vi "Grab images from pco.edge or pco.pixelfly USB.vi"() -> ()   [LabVIEW 2012]
doc: "A short program to demonstrate the fundamentals of control and image acquision with the pco.camera series. The program records a sequence of images, with \"live\" updating, until the \"StopRecording\" button is pressed. Use ctrl-H for more help on the individual controls and indicators.\n\nCopyright 2004, 2010 The Cooke Corporation."
panel:
  out "bClose":bool
  in  "Quit":bool
  out "BufNr1":i16
  out "BufNr0":i16
  in  "bUseBuffer1":bool
  in  "bUseBuffer0":bool
  in  "ROIX1":u16=1 min=1
  in  "ROIY1":u16=1 min=1
  in  "ROIY0":u16=1 min=1
  in  "ROIX0":u16=1 min=1
  out "Bits/pixel":u16
  in  "Record":bool
  in  "DelayTimeBase":u16(ring)=2 items=["nanoseconds", "microseconds", "milliseconds"]
  in  "ExposureTimeBase":u16(ring)=2 items=["nanoseconds", "microseconds", "milliseconds"]
  in  "Exposure":u32=10
  in  "Delay":u32
  in  "Rate":i32(ring) items=["12500000", "25000000"]
  out "Image":u16[][](graph)
  in  "TriggerMode":u16(ring) items=["Auto", "Software", "External sequence start ", "External exposure control"]
  # "A short program to demonstrate the fundamentals of control and image acquision with the pco.camera series. The program records a sequence of images, with \"live\" updating, until the \"StopRecording\" button is pressed.  Use ctrl-H for more help on the individual controls and indicators."
  # "pco.labview"
  # "1) Setup camera:"
  # "2) Record  images:"
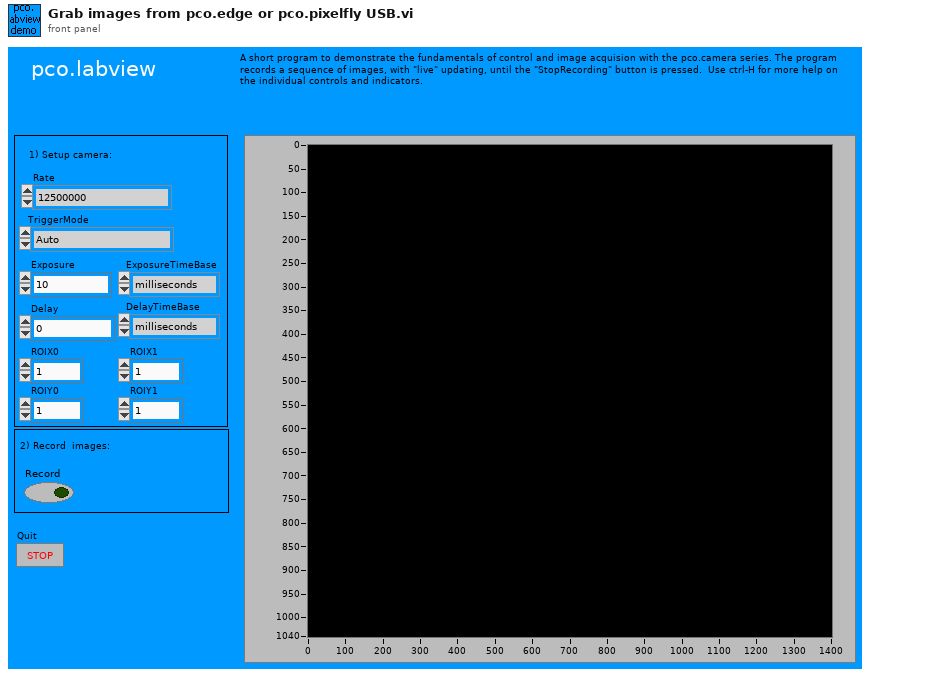
[diagram p1: front panel]
types:
  T1 = cluster{"SSize":u16, "CamType":u16, "CamsSubType":u16, "SerialNumber":u32, "HWVersion":u32, "FWVersion ":u32, "InterfaceType":u16, "HardwareVersions":cluster{"Board":u16, cluster{"string":string, "BatchNumber":u16, "MinorRevision":u8, "MajorRevision":u8, "Variant":u16}[]}, "FirmwareVersions":cluster{"DeviceNum":u16, cluster{"string":string, "MinorRevision":u8, "MajorRevision":u8, "Variant":u16}[]}}
  T2 = cluster{"Size":u16, "SensorTypeDESC":u16, "SensorSubtypeDESC":u16, "MaxHorizontalResStdDESC":u16, "MaxVerticalResStdDESC":u16, "MaxHorizontalResExtDESC":u16, "MaxVerticalResExtDESC":u16, "DynResDESC":u16, "MaxBinHorzDESC":u16, "BinHorzStepDESC":bool, "MaxBinVertDESC":u16, "BinVertStepDESC":bool, "ROIHorzStepDESC":u16, "ROIVertStepDESC":u16, "NumADCDESC":u16, "IRDESC":bool, "MinDelayDESC":u32, "MaxDelayDESC":u32, "MinDelayStepDESC":u32, "MinExpoDESC":u32, "MaxExpoDESC":u32, "MinExpoStepDESC":u32, "MinDelayIRDESC":u32, "MaxDelayIRDESC":u32, "MinExpoIRDESC":u32, "MaxExpoIRDESC":u32, "TimeTableDESC":bool, "DoubleImageDESC":bool, "MinCoolSetDESC":i16, "MaxCoolSetDESC":i16, "MDefaultCoolSetDESC":i16, "PowerDownModeDESC":bool, "OffsetRegDESC":bool, "ColorPattern":cluster{"UpperLeftColor":u8, "UpperRightColor":u8, "LowerLeftColor":u8, "LowerRightColor":u8}, "PatternTypeDESC":bool, "PixelRates":u32[], "CoversionFactors":u16[], "Reserved":u32[], "GeneralCapabilities":u32, "GeneralCapabilities 2":u32, "Min Size Hor":u16, "Min Size Vert":u16, "Ext Synch Freq":u32[], "Cooling Setpoints":i16[], "Soft ROI Hor Step":u16, "Soft ROI Vert Step":u16}
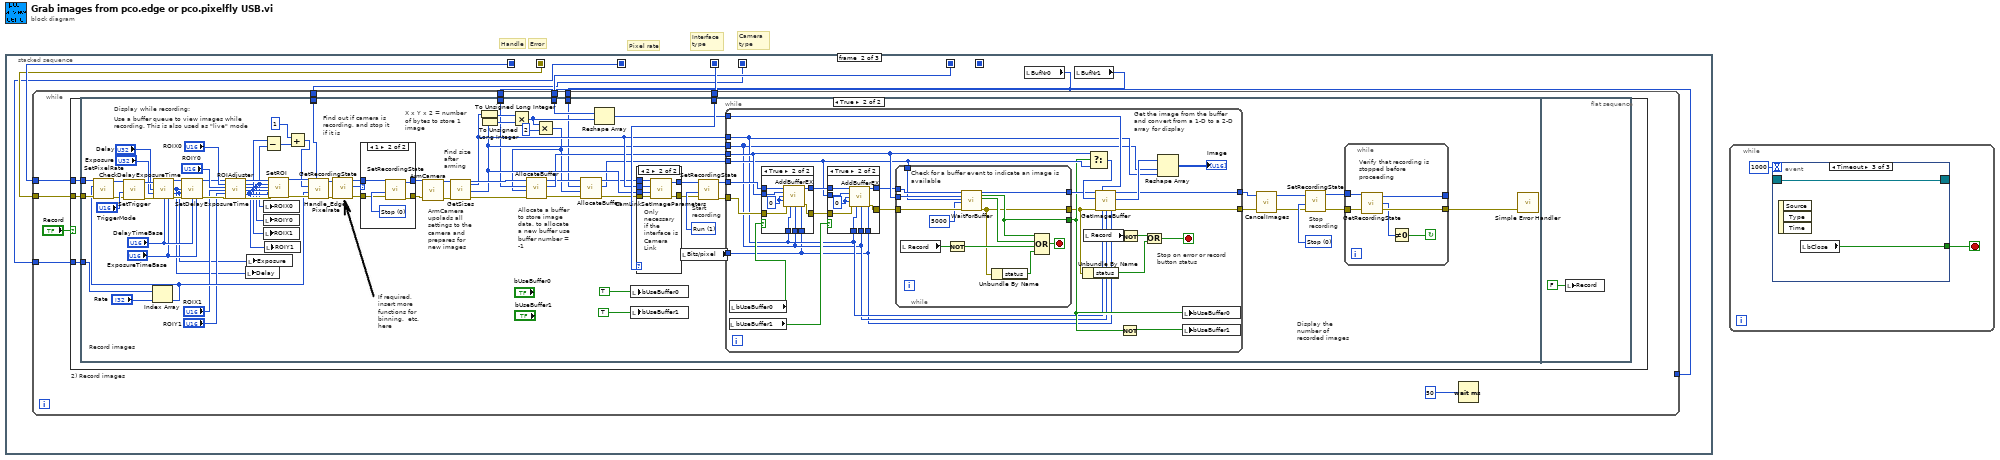
[diagram p0: block diagram]
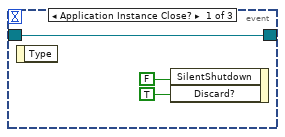
[diagram p2: hidden frame]
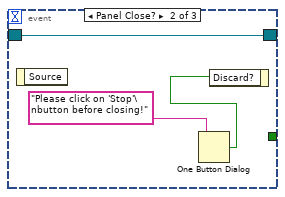
[diagram p3: hidden frame]
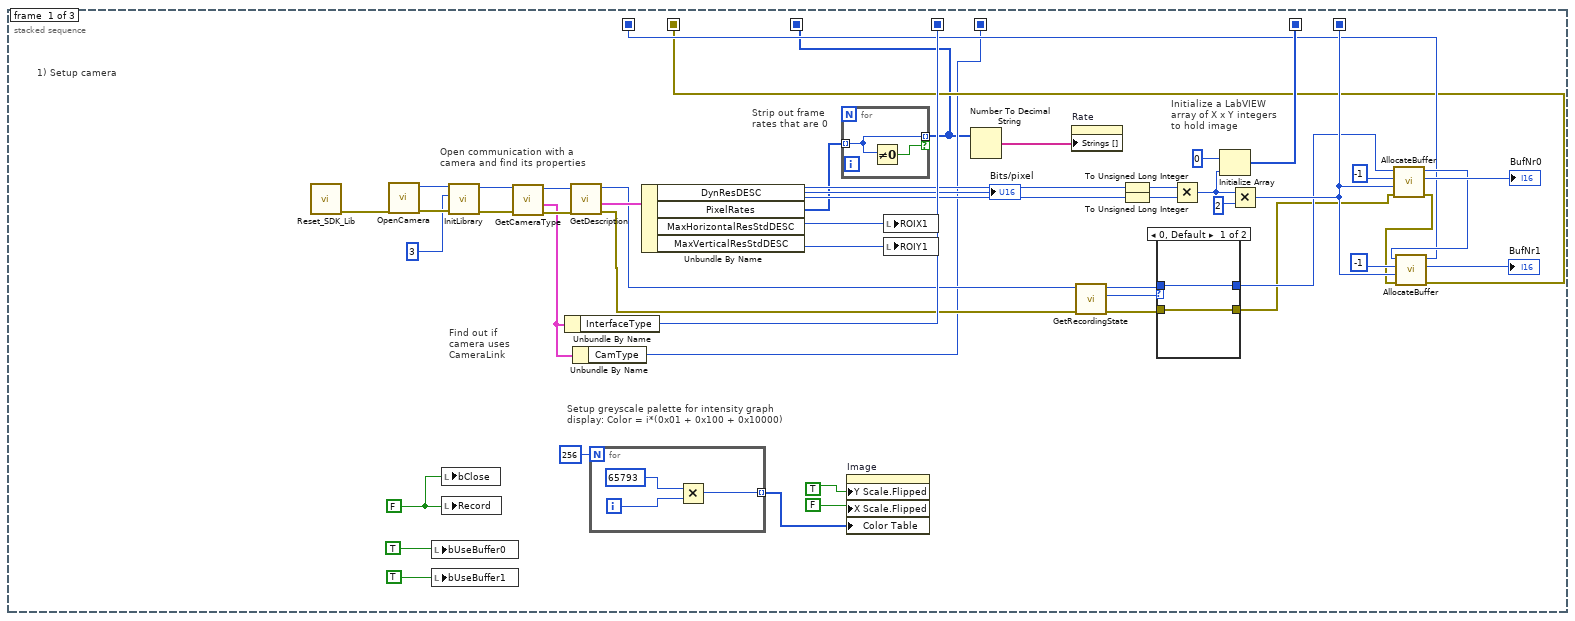
[diagram p4: hidden frame]
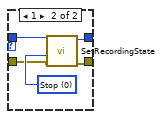
[diagram p5: hidden frame]
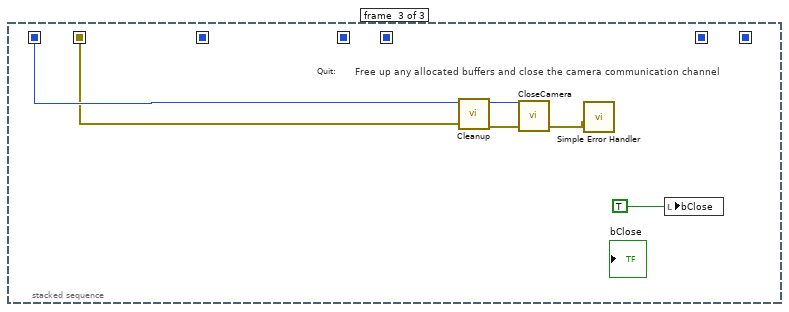
[diagram p11: hidden frame]
diagram:
  # "Camera type"
  # "Interface type"
  # "Error"
  # "Handle"
  # "Pixel rate"
  n1 = stacked-sequence {
    seq-local: [w41 _ _] -> [_ w64 _]
    seq-local: [w29 _ _] -> [_ _ _]
    seq-local: [w9 _ _] -> [_ w67 w253]
    seq-local: [w8 _ _] -> [_ w66 w252]
    seq-local: [w36 _ _] -> [_ w65 _]
    seq-local: [w1 _ _] -> [_ w61 _]
    seq-local: [w3 _ _] -> [_ w60 _]
    frame #0 {
      w23 = FALSE ("stop")
      # "Strip out frame rates that are 0"
      # "1) Setup camera"
      # "Find out if camera uses CameraLink"
      # "Setup greyscale palette for intensity graph display: Color = i*(0x01 + 0x100 + 0x10000)"
      # "Initialize a LabVIEW array of X x Y integers to hold image"
      # "Open communication with a camera and find its properties"
      n2 = call "Reset_SDK_Lib.vi"() -> ("ErrorOut"=w5:errorcluster)  [unwired: 11 in]
      n3 = call "OpenCamera.vi"("ErrorIn"=w5) -> ("ErrorOut"=w20:errorcluster, "Handle out"=w21:u64)  [unwired: 3 in, 2 out]
      n4 = local write "bUseBuffer0"(TRUE) -> ()
      n5 = local write "bUseBuffer1"(TRUE) -> ()
      n6 = local write "bClose"(w23) -> ()
      n7 = local write "Record"(w23) -> ()
      n8 = call "InitLibrary.vi"("error in (no error)"=w20, "InterfaceType"=u32 3, "ph"=w21) -> ("error out"=w19:errorcluster, "hout"=w18:u64)  [unwired: 7 in]
      n9 = call "GetCameraType.vi"("ph"=w18, "error in (no error)"=w19) -> ("hout"=w38:u64, "CameraType"=w4:T1, "error out"=w37:errorcluster)  [unwired: 1 in, 1 out]
      n10 = Unbundle By Name(w4) -> ("InterfaceType"=w36:u16)
      n11 = call "GetDescription.vi"("ErrorIn"=w37, "ph"=w38) -> ("ErrorOut"=w15:errorcluster, "Description"=w40:T2, "hout"=w14:u64)  [unwired: 2 in, 1 out]
      n12 = Unbundle By Name(w4) -> ("CamType"=w3:u16)
      n13 = for {
        N: 256 -> [_]
        tunnel: [w57] -> w44 mode=indexing
        i -> [w58]
        n14 = Multiply(x=65793, y=w58) -> (x*y=w57:i32)
      }
      n15 = Unbundle By Name(w40) -> ("DynResDESC"=→"Bits/pixel":u16, "PixelRates"=w2:u32[], "MaxHorizontalResStdDESC"=w34:u16, "MaxVerticalResStdDESC"=w33:u16)
      n16 = for {
        tunnel: w2 -> [w48] mode=indexing
        tunnel: [w48] -> w1 mode=indexing if=w49
        n17 = Not Equal To 0?(x=w48) -> (x != 0?=w49:bool)
      }
      n18 = property on="Image" class="IntGraph (strict)"("Y Scale.Flipped"=TRUE, "X Scale.Flipped"=FALSE, "Color Table"=w44) -> ()  [unwired: 2 in, 2 out]
      n19 = local write "ROIX1"(w34) -> ()
      n20 = local write "ROIY1"(w33) -> ()
      n21 = Number To Decimal String(number=w1) -> (decimal integer string=w22:string[])  [unwired: 1 in]
      n22 = property on="Rate" class="Ring (strict)"("Strings []"=w22) -> ()  [unwired: 2 in, 2 out]
      n23 = call "GetRecordingState.vi"("ErrorIn"=w15, "ph"=w14) -> ("ErrorOut"=w12:errorcluster, "Error"=w6:i32, "hout"=w13:u64)  [unwired: 2 in, 1 out]
      n24 = To Unsigned Long Integer(number=w34) -> (unsigned 32bit integer=w31:u32)
      n25 = To Unsigned Long Integer(number=w33) -> (unsigned 32bit integer=w30:u32)
      n26 = case shown="0, Default" w6 {
        tunnel: w13 -> [w51 w55]
        tunnel: w12 -> [w50 w54]
        tunnel: [w51 w53] -> w11
        tunnel: [w50 w52] -> w7
        frame 0, Default {
        }
        frame 1 {
          w56 = u16 0 items=["Stop", "Run"] ("RecordingState")
          n27 = call "SetRecordingState.vi"("ErrorIn"=w54, "RecordingState"=w56, "ph"=w55) -> ("ErrorOut"=w52:errorcluster, "hout"=w53:u64)  [unwired: 2 in, 1 out]
        }
      }
      n28 = Multiply(x=w31, y=w30) -> (x*y=w42:u32)
      n29 = Initialize Array(u16 0 ("Element Data"), w42) -> (w41:u16[])
      n30 = Multiply(x=w42, y=u32 2) -> (x*y=w29:u32)
      n31 = call "AllocateBuffer.vi"("error in (no error)"=w7, "Size"=w29, "BufNr"=i16 -1, "ph"=w11) -> ("error out"=w16:errorcluster, "BufNrOut"=→"BufNr0":i16, "hout"=w10:u64)  [unwired: 2 in, 3 out]
      n32 = call "AllocateBuffer.vi"("error in (no error)"=w16, "Size"=w29, "BufNr"=i16 -1, "ph"=w10) -> ("error out"=w8:errorcluster, "BufNrOut"=→"BufNr1":i16, "hout"=w9:u64)  [unwired: 2 in, 3 out]
    }
    frame #1 {
      n33 = local read "BufNr0"() -> (w63:i16)
      n34 = local read "BufNr1"() -> (w62:i16)
      n35 = while {
        tunnel: w63 -> [_]
        tunnel: w63 -> [w73]
        tunnel: w64 -> [w75]
        tunnel: w65 -> [w76]
        tunnel: w66 -> [w74]
        tunnel: w67 -> [w71]
        tunnel: w62 -> [w72]
        tunnel: w61 -> [w69]
        tunnel: w60 -> [w68]
        stop <- "Quit" stop-if-true
        n36 = case "2) Record images" shown="True" "Record" {
          tunnel: w71 -> [_ w86]
          tunnel: w74 -> [_ w85]
          tunnel: w76 -> [_ w84]
          tunnel: w75 -> [_ w83]
          tunnel: w73 -> [_ w82]
          tunnel: w72 -> [_ w81]
          tunnel: w69 -> [_ w80]
          tunnel: w68 -> [_ w79]
          frame False {
          }
          frame True {
            n37 = flat-sequence {
              tunnel: w86 -> [w151]
              tunnel: w85 -> [w150]
              tunnel: w84 -> [w148]
              tunnel: w83 -> [w146]
              tunnel: w82 -> [w137]
              tunnel: w81 -> [w131]
              tunnel: w80 -> [w118]
              tunnel: w79 -> [w109]
              frame #0 {
                w164 = u16 1 items=["Stop", "Run"] ("RecordingState")
                w167 = u16 0 items=["Stop", "Run"] ("RecordingState")
                # "Display the number of recorded images"
                # "Record images"
                # "Start recording"
                # "Allocate a buffer to store image data. to allocate a new buffer use buffer number = -1"
                # "Find size after arming"
                # "ArmCamera upolads all settings to the camera and prepares for new images"
                # "Find out if camera is recording, and stop it if it is"
                # "If required, insert more functions for binning.  etc. here"
                # "X x Y x 2 = number of bytes to store 1 image"
                # "Stop recording"
                # "Use a buffer queue to view images while recording. This is also used as \"live\" mode"
                # "Display while recording:"
                n38 = Index Array(array=w118, index="Rate") -> (element=w113:u32)
                n39 = call "SetPixelRate.vi"("error in (no error)"=w150, "PixelRate"=w113, "ph"=w151) -> ("error out"=w120:errorcluster, "hout"=w121:u64)  [unwired: 2 in, 1 out]
                n40 = call "SetTrigger.vi"("error in (no error)"=w120, "TriggerMode"="TriggerMode", "ph"=w121) -> ("error out"=w94:errorcluster, "hout"=w96:u64)  [unwired: 2 in, 1 out]
                n41 = call "CheckDelayExposureTime.vi"("ph"=w96, "Delay"="Delay", "Exposure"="Exposure", "error in (no error)"=w94, "DelayTimeBase"="DelayTimeBase", "ExposureTimeBase"="ExposureTimeBase") -> ("hout"=w95:u64, "Delay Out"=w88:u32, "Exposure Out"=w87:u32, "error out"=w89:errorcluster)  [unwired: 4 in, 2 out]
                n42 = call "SetDelayExposureTime.vi"("ph"=w95, "Delay"=w88, "Exposure"=w87, "error in (no error)"=w89, "DelayTimeBase"="DelayTimeBase", "ExposureTimeBase"="ExposureTimeBase") -> ("hout"=w102:u64, "error out"=w108:errorcluster)  [unwired: 7 in, 1 out]
                n43 = call "ROIAdjuster.vi"("HandleIn"=w102, "ROIXmin"="ROIX0", "ROIYmin"="ROIY0", "ROIXmax"="ROIX1", "ROIYmax"="ROIY1", "ErrorIn"=w108) -> ("hout"=w101:u64, "ROIX0Mod"=w97:u16, "ROIY0Mod"=w98:u16, "ROIX1Mod"=w99:u16, "ROIY1Mod"=w100:u16, "ErrorOut"=w107:errorcluster)  [unwired: 7 in, 1 out]
                n44 = local write "Delay"(w88) -> ()
                n45 = local write "Exposure"(w87) -> ()
                n46 = Subtract(x=w99, y=w97) -> (x-y=w112:u16)
                n47 = local write "ROIX0"(w97) -> ()
                n48 = local write "ROIY0"(w98) -> ()
                n49 = local write "ROIX1"(w99) -> ()
                n50 = local write "ROIY1"(w100) -> ()
                n51 = call "SetROI.vi"("ph"=w101, "ROIX0"=w97, "ROIY0"=w98, "ROIX1"=w99, "ROIY1"=w100, "error in (no error)"=w107) -> ("hout"=w114:u64, "error out"=w115:errorcluster)  [unwired: 12 in]
                n52 = Add(x=1, y=w112) -> (x+y=w110:i32)
                n53 = call "Handle_Edge_Pixelrate.vi"("Cameratype"=w109, "error in (no error)"=w115, "PixelRate"=w113, "X-Resolution"=w110, "ph"=w114) -> ("error out"=w116:errorcluster, "hout"=w117:u64)  [unwired: 5 in]
                n54 = call "GetRecordingState.vi"("ErrorIn"=w116, "ph"=w117) -> ("ErrorOut"=w161:errorcluster, "RecordingState"=w163:u16, "hout"=w162:u64)  [unwired: 2 in, 1 out]
                n55 = case shown="1" w163 {
                  tunnel: w162 -> [w245 w249]
                  tunnel: w161 -> [w244 w248]
                  tunnel: [w245 w247] -> w160
                  tunnel: [w244 w246] -> w159
                  frame 0, Default {
                  }
                  frame 1 {
                    w250 = u16 0 items=["Stop", "Run"] ("RecordingState")
                    n56 = call "SetRecordingState.vi"("ErrorIn"=w248, "RecordingState"=w250, "ph"=w249) -> ("ErrorOut"=w246:errorcluster, "hout"=w247:u64)  [unwired: 2 in, 1 out]
                  }
                }
                n57 = call "ArmCamera.vi"("error in (no error)"=w159, "ph"=w160) -> ("error out"=w157:errorcluster, "hout"=w158:u64)  [unwired: 1 in, 1 out]
                n58 = call "GetSizes.vi"("ph"=w158, "ErrorIn"=w157) -> ("hout"=w154:u64, "XResAct"=w144:u16, "YResAct"=w143:u16, "ErrorOut"=w156:errorcluster)  [unwired: 11 in, 3 out]
                n59 = To Unsigned Long Integer(number=w144) -> (unsigned 32bit integer=w138:u32)
                n60 = To Unsigned Long Integer(number=w143) -> (unsigned 32bit integer=w139:u32)
                n61 = Multiply(x=w138, y=w139) -> (x*y=w140:u32)
                n62 = Multiply(x=w140, y=u32 2) -> (x*y=w132:u32)
                n63 = call "AllocateBuffer.vi"("error in (no error)"=w156, "Size"=w132, "BufNr"=w137, "ph"=w154) -> ("error out"=w136:errorcluster, "BufNrOut"=w141:i16, "hout"=w134:u64)  [unwired: 2 in, 3 out]
                n64 = call "AllocateBuffer.vi"("error in (no error)"=w136, "Size"=w132, "BufNr"=w131, "ph"=w134) -> ("error out"=w135:errorcluster, "BufNrOut"=w130:i16, "hout"=w133:u64)  [unwired: 2 in, 3 out]
                n65 = Reshape Array(w146, w140) -> (w145:u16[])
                n66 = local write "bUseBuffer0"(TRUE) -> ()
                n67 = local write "bUseBuffer1"(TRUE) -> ()
                n68 = case shown="2" w148 {
                  tunnel: w135 -> [w236 w243]
                  tunnel: [w236 w242] -> w153
                  tunnel: w133 -> [w237 w241]
                  tunnel: [w237 w240] -> w152
                  tunnel: w143 -> [_ w239]
                  tunnel: w144 -> [_ w238]
                  frame 0, Default {
                  }
                  frame 2 {
                    # "Only necessary if the interface is Camera Link"
                    n69 = call "CamLinkSetImageParameters.vi"("error in (no error)"=w243, "YRes"=w239, "XRes"=w238, "ph"=w241) -> ("error out"=w242:errorcluster, "hout"=w240:u64)  [unwired: 1 out]
                  }
                }
                n70 = local read "Bits/pixel"() -> (w125:u16)
                n71 = call "SetRecordingState.vi"("ErrorIn"=w153, "RecordingState"=w164, "ph"=w152) -> ("ErrorOut"=w149:errorcluster, "hout"=w147:u64)  [unwired: 2 in, 1 out]
                n72 = while {
                  tunnel: w141 -> [w180]
                  tunnel: w145 -> [w190]
                  tunnel: w147 -> [w189]
                  tunnel: w143 -> [w169]
                  tunnel: w144 -> [w170]
                  tunnel: w149 -> [w187]
                  tunnel: [w192] -> w124
                  tunnel: [w193] -> w123
                  tunnel: w130 -> [w179]
                  tunnel: w125 -> [w168]
                  stop <- w171 stop-if-true
                  # "Stop on error or record button status"
                  # "Get the image from the buffer and convert from a 1-D to a 2-D array for display"
                  n73 = local read "bUseBuffer1"() -> (w184:bool)
                  n74 = local read "bUseBuffer0"() -> (w185:bool)
                  n75 = case shown="True" w185 {
                    tunnel: [w196 w205] -> w186
                    tunnel: [w195 w204] -> w188
                    tunnel: w180 -> [_ w203]
                    tunnel: w189 -> [w195 w202]
                    tunnel: w168 -> [_ w200]
                    tunnel: w170 -> [_ w199]
                    tunnel: w169 -> [_ w198]
                    tunnel: w187 -> [w196 w197]
                    frame False {
                    }
                    frame True {
                      w201 = i16 0
                      n76 = call "AddBufferEX.vi"("ph"=w202, "BuffNr"=w203, "1stImage"=w201, "LastImage"=w201, "error in (no error)"=w197, "XRes"=w199, "YRes"=w198, "BitPerPixel"=w200) -> ("hout"=w204:u64, "error out"=w205:errorcluster)  [unwired: 5 in, 1 out]
                    }
                  }
                  n77 = case shown="True" w184 {
                    tunnel: [w206 w216] -> w177
                    tunnel: [w207 w215] -> w178
                    tunnel: w179 -> [_ w214]
                    tunnel: w188 -> [w207 w213]
                    tunnel: w168 -> [_ w211]
                    tunnel: w170 -> [_ w210]
                    tunnel: w169 -> [_ w209]
                    tunnel: w186 -> [w206 w208]
                    frame False {
                    }
                    frame True {
                      w212 = i16 0
                      n78 = call "AddBufferEX.vi"("ph"=w213, "BuffNr"=w214, "1stImage"=w212, "LastImage"=w212, "error in (no error)"=w208, "XRes"=w210, "YRes"=w209, "BitPerPixel"=w211) -> ("hout"=w215:u64, "error out"=w216:errorcluster)  [unwired: 5 in, 1 out]
                    }
                  }
                  n79 = while {
                    tunnel: w180 -> [w224]
                    tunnel: w179 -> [w223]
                    tunnel: w178 -> [w226]
                    tunnel: w177 -> [w225]
                    tunnel: [w222] -> w176
                    tunnel: [w218] -> w174
                    tunnel: [w221] -> w175
                    stop <- w227 stop-if-true
                    # "Check for a buffer event to indicate an image is available"
                    n80 = local read "Record"() -> (w229:bool)
                    n81 = Not(x=w229) -> (.not. x?=w228:bool)
                    n82 = call "WaitForBuffer.vi"("ph"=w226, "sBufNr"=w224, "sBufNr 2"=w223, "timeout"=5000, "error in (no error)"=w225) -> ("hout"=w222:u64, "Buffer_Ready"=w221:bool, "Buffer_Ready 2"=w220:bool, "error out"=w218:errorcluster)  [unwired: 10 in, 1 out]
                    n83 = Unbundle By Name(w218) -> ("status"=w217:bool)
                    n84 = Compound Arithmetic op=OR(w221, w220, w228, w217) -> (w227:bool)
                  }
                  n85 = Unbundle By Name(w174) -> ("status"=w172:bool)
                  n86 = local read "Record"() -> (w191:bool)
                  n87 = Select(t=w180, s=w175, f=w179) -> (s? t:f=w183:i16)
                  n88 = call "GetImageBuffer.vi"("ph"=w176, "BuffIn"=w190, "BuffNr"=w183, "error in (no error)"=w174, "xRes"=w170, "yRes"=w169, "Bitresolution"=w168) -> ("hout"=w192:u64, "BuffOut"=w194:u16[], "error out"=w193:errorcluster)  [unwired: 5 in, 1 out]
                  n89 = Not(x=w175) -> (.not. x?=w182:bool)
                  n90 = Not(x=w191) -> (.not. x?=w173:bool)
                  n91 = Or(x=w173, y=w172) -> (x .or. y?=w171:bool)
                  n92 = Reshape Array(w194, w169, w170) -> (→"Image":u16[][])
                  n93 = local write "bUseBuffer0"(w175) -> ()
                  n94 = local write "bUseBuffer1"(w182) -> ()
                }
                n95 = call "CancelImages.vi"("error in (no error)"=w123, "ph"=w124) -> ("error out"=w127:errorcluster, "hout"=w126:u64)  [unwired: 1 in, 1 out]
                n96 = call "SetRecordingState.vi"("ErrorIn"=w127, "RecordingState"=w167, "ph"=w126) -> ("ErrorOut"=w165:errorcluster, "hout"=w166:u64)  [unwired: 2 in, 1 out]
                n97 = while {
                  tunnel: [w233] -> w122
                  tunnel: w165 -> [w234]
                  tunnel: w166 -> [w235]
                  tunnel: [w230] -> _
                  stop <- w231 continue-if-true
                  # "Verify that recording is stopped before proceeding"
                  n98 = call "GetRecordingState.vi"("ErrorIn"=w234, "ph"=w235) -> ("ErrorOut"=w233:errorcluster, "RecordingState"=w232:u16, "hout"=w230:u64)  [unwired: 2 in, 1 out]
                  n99 = Not Equal To 0?(x=w232) -> (x != 0?=w231:bool)
                }
                n100 = call <vilib>:"Simple Error Handler.vi"("error in (no error)"=w122) -> ()  [unwired: 4 in, 5 out]
              }
              frame #1 {
                n101 = local write "Record"(FALSE ("Record")) -> ()
              }
            }
          }
        }
        n102 = Wait (ms)(milliseconds to wait=u32 50) -> ()  [unwired: 1 out]
      }
    }
    frame #2 {
      # "Free up any allocated buffers and close the camera communication channel"
      # "Quit:"
      n103 = call "Cleanup.vi"("error in (no error)"=w252, "ph"=w253) -> ("error out"=w254:errorcluster, "hout"=w255:u64)  [unwired: 8 in]
      n104 = call "CloseCamera.vi"("ErrorIn"=w254, "Handle in"=w255) -> ("ErrorOut"=w257:errorcluster)  [unwired: 1 in, 2 out]
      n105 = call <vilib>:"Simple Error Handler.vi"("error in (no error)"=w257) -> ()  [unwired: 4 in, 5 out]
      n106 = local write "bClose"(TRUE) -> ()
    }
  }
  n107 = while {
    stop <- w258 stop-if-true
    n108 = event shown="[2] Timeout" {
      selector: _ -> [w260 w265 w267]
      dyn-events: [w260 w265 w267] -> _
      timeout: 1000 -> [_ _ _]
      tunnel: [_ _ w266] -> w258
      event Application Instance Close? {
        n109 = event-data() -> ()  [unwired: 1 in, 1 out]
        n110 = event-data("SilentShutdown"=FALSE, "Discard?"=TRUE) -> ()  [unwired: 1 in, 1 out]
      }
      event Panel Close? {
        n111 = event-data() -> ()  [unwired: 1 in, 1 out]
        n112 = One Button Dialog(message="Please click on 'Stop'\nbutton before closing!") -> (true=w263:bool)  [unwired: 1 in]
        n113 = event-data("Discard?"=w263) -> ()  [unwired: 1 in, 1 out]
      }
      event Timeout {
        n114 = event-data() -> ()  [unwired: 1 in, 3 out]
        n115 = local read "bClose"() -> (w266:bool)
      }
    }
  }
